vi "Decoder.vi"() -> ()   [LabVIEW 2020]
panel:
  out "Y3":bool
  out "Y2":bool
  out "Y1":bool
  out "Y0":bool
  in  "EN":bool
  in  "B":bool
  in  "A":bool
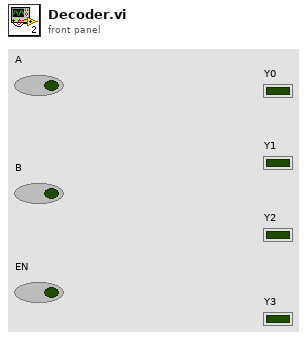
[diagram p1: front panel]
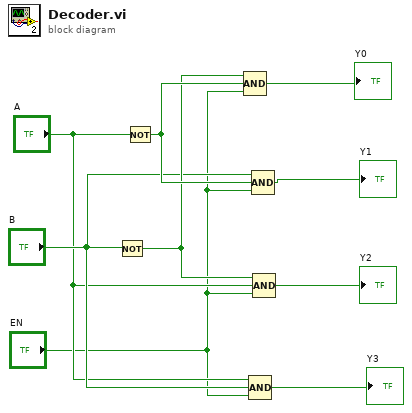
[diagram p0: block diagram]
diagram:
  n1 = Not(x="B") -> (.not. x?=w4:bool)
  n2 = Not(x="A") -> (.not. x?=w5:bool)
  n3 = Compound Arithmetic op=AND(w4, w5, "EN") -> (→"Y0":bool)
  n4 = Compound Arithmetic op=AND("A", "B", "EN") -> (→"Y3":bool)
  n5 = Compound Arithmetic op=AND("B", w5, "EN") -> (→"Y1":bool)
  n6 = Compound Arithmetic op=AND(w4, "A", "EN") -> (→"Y2":bool)
